vi "ELVIS III v1.0 Reserve AO.vi"(7 "Allow multiple opens?":bool, 8 "error in (no error)":errorcluster, 10 "AO Channel List":T1) -> (0 "error out":errorcluster)   [LabVIEW 2021]
uses:
  <vilib>/myRIO/Common/Instrument Driver Framework/myRIO v1.0/AO/typedefs/AO Channels List.ctl
  <vilib>/myRIO/Common/Instrument Driver Framework/myRIO v1.0/AO/typedefs/AO Channels Enum.ctl
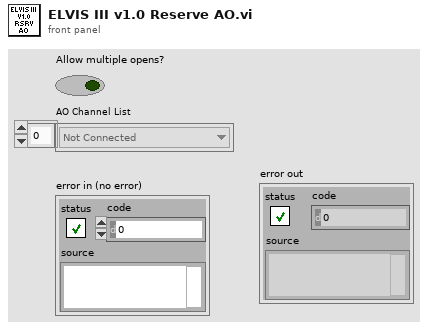
[diagram p1: front panel]
types:
  T1 = typedef "AO Channels List.ctl" = T2[]
  T2 = typedef "AO Channels Enum.ctl" = enum16{"Not Connected", "AudioOut/Left", "AudioOut/Right", "C/AO0", "C/AO1", "A/AO0", "A/AO1", "B/AO0", "B/AO1"}
  T3 = typedef "ELVIS III v1.0 Channel Reservation List.ctl" = T4[]
  T4 = typedef "ELVIS III v1.0 Channel Reservation Info.ctl" = cluster{"Channel Name":string, "Connector":T5, "MutexIDs":u32[]}
  T5 = typedef "ELVIS III v1.0 Connector List.ctl" = enum32{"None", "ConnectorA", "ConnectorB"}
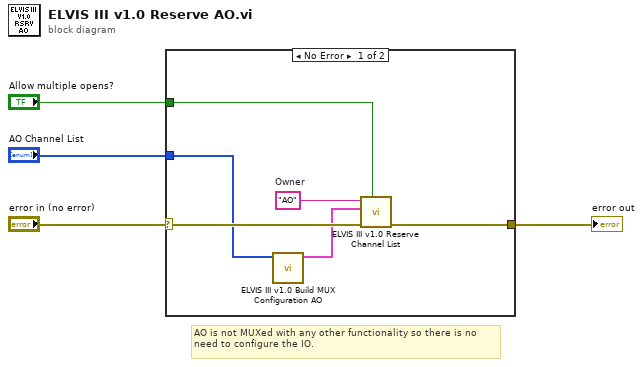
[diagram p0: block diagram]
diagram:
  # "AO is not MUXed with any other functionality so there is no need to configure the IO."
  n1 = case shown="No Error" "error in (no error)" {
    selector: "error in (no error)" -> [w9 w11]
    tunnel: "Allow multiple opens?" -> [w10 _]
    tunnel: "AO Channel List" -> [w7 _]
    tunnel: [w8 w11] -> w3
    frame No Error {
      w5 = "AO"  # Owner
      n2 = call <vilib>:"ELVIS III v1.0 Build MUX Configuration AO.vi"("AO Channels List"=w7) -> ("Channel Reservation Info"=w6:T3)  [unwired: 10 in]
      n3 = call <vilib>:"ELVIS III v1.0 Reserve Channel List.vi"("Allow multiple opens?"=w10, "error in (no error)"=w9, "Channel Reservation List"=w6, "Owner"=w5) -> ("error out"=w8:errorcluster)  [unwired: 7 in]
    }
    frame Error {
      # "There is an incoming error so there is nothing to do."
    }
  }
  "error out" <- w3
